vi "Close.vi"(8 "error in (no error)":errorcluster, 11 "NHRDCPower in":refnum<class "NHRDCPower.lvclass">) -> (0 "error out":errorcluster, 3 "NHRDCPower out":refnum<class "NHRDCPower.lvclass">)   [LabVIEW 2018, in "AcPwrPlugins.lvlib" / "NHRDCPower.lvclass"]
doc: "This VI closes the reference to the instrument(s)."
uses:
  NHRDCPower.lvclass
  <instrlib>/NHRDCPowerModule/NHRDCPowerModule/NHRDCPowerModule.lvlib
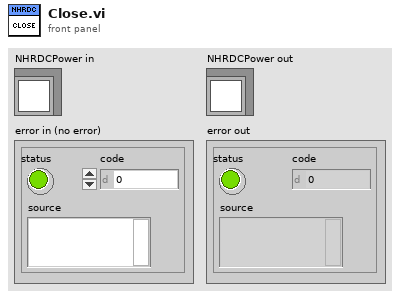
[diagram p1: front panel]
types:
  T1 = typedef "AcPwrPlugins.lvlib/NHRDCPower.lvclass/Device(s)Settings.ctl" = cluster{"MeasName":string, "Modules":T2}
  T2 = typedef "AcPwrPlugins.lvlib/NHRDCPower.lvclass/Modules.ctl" = cluster{"Handle":string, "Name":string, "id query (Yes)":bool, "reset device (Yes)":bool, "Connected":bool, "Initial Battery Detect Voltage (0)":sgl, "SafetySettings":cluster{"SetWatchDog?":bool, "Voltage (V)":sgl, "Current (A)":sgl, "Power (W)":sgl, "Voltage Delay (s)":sgl, "Current Delay (s)":sgl, "Power Delay (s)":sgl}, "Options String":string, "Aperture Time (s)":sgl, "operating state (Off)":i32, "OutputSettings":cluster{"Voltage (V)":sgl, "Current (A)":sgl, "Resistance (Ohms)":sgl, "Power (W)":sgl, "Enable Voltage":bool, "Enable Current":bool, "Enable Resistance":bool, "Enable Power":bool, "Macro After Step Delay  (s)":sgl, "Wait Value (V, A, W)":sgl, "Enable Wait":bool, "Wait on Value":i32}[], "SlewRate":cluster{"Set Voltage Rate V/S":dbl, "Set Current Rate A/S":dbl, "Set Resistance Rate R/S":dbl, "Set Power Rate W/S":dbl}, "Macro":cluster{"Save Macro?":bool, "Load Macro From File?":bool, "Run Macro Continuously?":bool, "Load Macro File Path":path, "Save Macro File Path":path, "Use Macros?":bool}}[]
  T3 = typedef "AcPwrPlugins.lvlib/NHRDCPower.lvclass/Measurements.ctl" = cluster{"Handle":string, "Name":string, "Enabled":bool, "Measurement Value":sgl, "btnMeasFetch":bool, "Measurement Type":i32, "Fetch Method":i32, "Fetch Time (s)":sgl}[]
  T4 = cluster{"Handle":string, "Name":string, "id query (Yes)":bool, "reset device (Yes)":bool, "Connected":bool, "Initial Battery Detect Voltage (0)":sgl, "SafetySettings":cluster{"SetWatchDog?":bool, "Voltage (V)":sgl, "Current (A)":sgl, "Power (W)":sgl, "Voltage Delay (s)":sgl, "Current Delay (s)":sgl, "Power Delay (s)":sgl}, "Options String":string, "Aperture Time (s)":sgl, "operating state (Off)":i32, "OutputSettings":cluster{"Voltage (V)":sgl, "Current (A)":sgl, "Resistance (Ohms)":sgl, "Power (W)":sgl, "Enable Voltage":bool, "Enable Current":bool, "Enable Resistance":bool, "Enable Power":bool, "Macro After Step Delay  (s)":sgl, "Wait Value (V, A, W)":sgl, "Enable Wait":bool, "Wait on Value":i32}[], "SlewRate":cluster{"Set Voltage Rate V/S":dbl, "Set Current Rate A/S":dbl, "Set Resistance Rate R/S":dbl, "Set Power Rate W/S":dbl}, "Macro":cluster{"Save Macro?":bool, "Load Macro From File?":bool, "Run Macro Continuously?":bool, "Load Macro File Path":path, "Save Macro File Path":path, "Use Macros?":bool}}
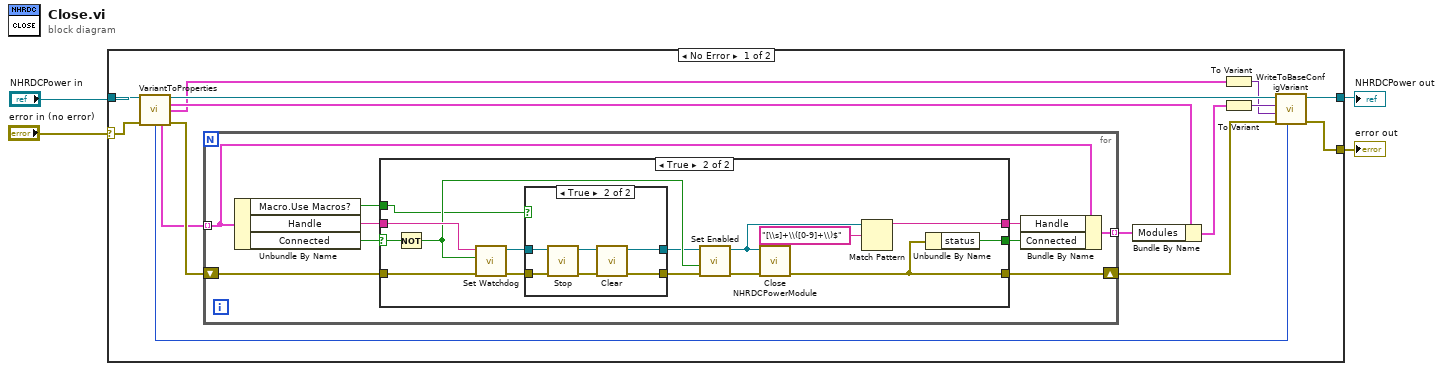
[diagram p0: block diagram]
diagram:
  n1 = case shown="No Error" "error in (no error)" {
    selector: "error in (no error)" -> [w14 w55]
    tunnel: [w18 w56] -> w2
    tunnel: "NHRDCPower in" -> [w15 w56]
    tunnel: [w17 w55] -> w1
    frame No Error {
      n2 = call "VariantToProperties.vi"("NHRDCPower in"=w15, "error in (no error)"=w14) -> ("NHRDCPower out"=w13:refnum<class "NHRDCPower.lvclass">, "NHRDC"=w8:T1, "Meas"=w5:T3, "Measurement Refresh Time (ms)"=w7:u32, "Modules"=w11:T2, "error out"=w12:errorcluster)  [unwired: 7 in, 1 out]
      n3 = for {
        tunnel: w11 -> [w28] mode=indexing
        shift-right: [w26] -> w16
        shift-left: w12 -> [w27]
        tunnel: [w25] -> w9 mode=indexing
        n4 = Unbundle By Name(w28) -> ("Macro.Use Macros?"=w20:bool, "Handle"=w24:string, "Connected"=w21:bool)
        n5 = case shown="True" w21 {
          selector: w21 -> [w29 w40]
          tunnel: w24 -> [w30 w41]
          tunnel: w27 -> [w31 w44]
          tunnel: [w31 w43] -> w26
          tunnel: [w30 w45] -> w23
          tunnel: [w29 w42] -> w22
          tunnel: w20 -> [_ w32]
          frame False {
          }
          frame True {
            n6 = Not(x=w40) -> (.not. x?=w37:bool)
            n7 = call <instrlib>:"Set Watchdog.vi"("error in (no error)"=w44, "watchdog"=w37, "instrument handle"=w41) -> ("error out"=w36:errorcluster, "instrument handle out"=w34:refnum<visa-resource-name>)  [unwired: 7 in]
            n8 = case shown="True" w32 {
              tunnel: w36 -> [w48 w54]
              tunnel: [w48 w49] -> w35
              tunnel: w34 -> [w47 w53]
              tunnel: [w47 w50] -> w33
              frame False {
              }
              frame True {
                n9 = call <instrlib>:"Stop.vi"("error in (no error)"=w54, "instrument handle"=w53) -> ("error out"=w52:errorcluster, "instrument handle out"=w51:refnum<visa-resource-name>)  [unwired: 8 in]
                n10 = call <instrlib>:"Clear.vi"("error in (no error)"=w52, "instrument handle"=w51) -> ("error out"=w49:errorcluster, "instrument handle out"=w50:refnum<visa-resource-name>)  [unwired: 8 in]
              }
            }
            n11 = call <instrlib>:"Set Enabled.vi"("error in (no error)"=w35, "enabled (false)"=w37, "instrument handle"=w33) -> ("error out"=w39:errorcluster, "instrument handle out"=w38:refnum<visa-resource-name>)  [unwired: 7 in]
            n12 = call <instrlib>:"Close NHRDCPowerModule.vi"("error in (no error)"=w39, "instrument handle"=w38) -> ("error out"=w43:errorcluster)  [unwired: 9 in]
            n13 = Match Pattern(string=w38, regular expression="[\\s]+\\([0-9]+\\)$") -> (before substring=w45:string)  [unwired: 1 in, 3 out]
            n14 = Unbundle By Name(w43) -> ("status"=w42:bool)
          }
        }
        n15 = Bundle By Name(cluster=w28, "Handle"=w23, "Connected"=w22) -> (w25:T4)
      }
      n16 = Bundle By Name(cluster=w8, "Modules"=w9) -> (w10:T1)
      n17 = To Variant(anything=w5) -> (Variant=w6:variant)
      n18 = To Variant(anything=w10) -> (Variant=w19:variant)
      n19 = call "WriteToBaseConfigVariant.vi"("Measurement Refresh Time (ms)"=w7, "error in (no error)"=w16, "Meas"=w6, "Config"=w19, "NHRDCPower in"=w13) -> ("error out"=w17:errorcluster, "NHRDCPower out"=w18:refnum<class "NHRDCPower.lvclass">)  [unwired: 5 in]
    }
    frame Error {
    }
  }
  "error out" <- w1
  "NHRDCPower out" <- w2
